vi "Arm Sensors OK.vi"(1 "Motor In":dbl, 2 "Pot Angle":dbl, 3 "Encoder Angle":dbl, 4 "Pot Voltage":dbl) -> (0 "Motor Out":dbl)   [LabVIEW 2013]
uses:
  Robot Global Data.vi
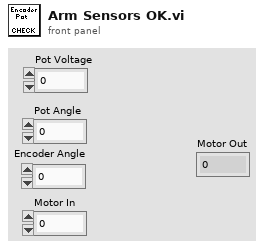
[diagram p1: front panel]
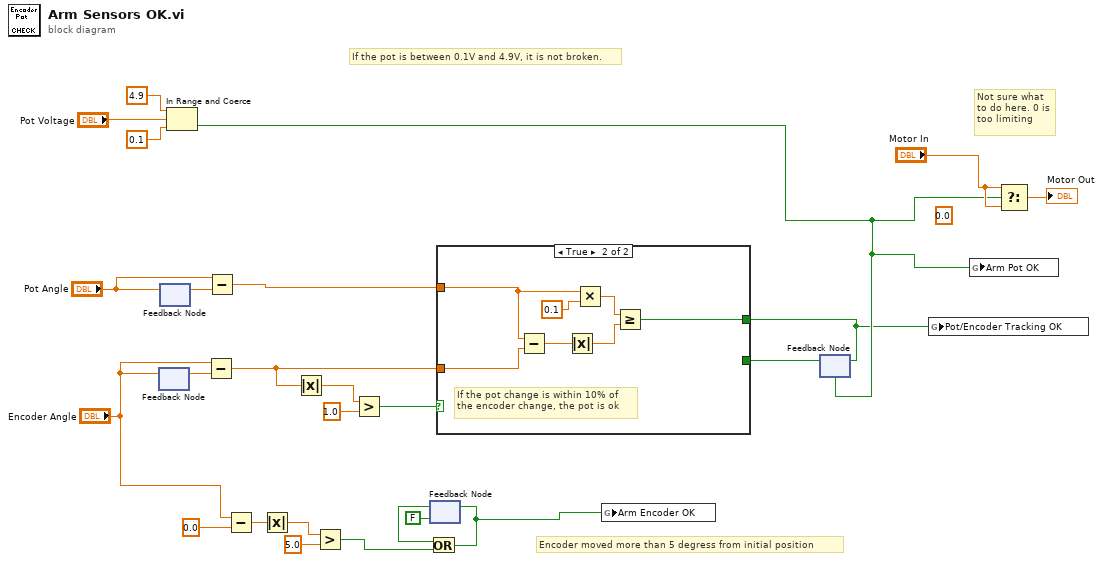
[diagram p0: block diagram]
diagram:
  (unwired) 0.0 ("f")
  # "Not sure what\nto do here. 0 is\ntoo limiting"
  # "Encoder moved more than 5 degress from initial position"
  # "If the pot is between 0.1V and 4.9V, it is not broken."
  n1 = feedback #1() -> (w23:dbl)  [unwired: 1 in]
  n2 = feedback-in #1("Encoder Angle") -> ()
  n3 = feedback #2() -> (w24:dbl)  [unwired: 1 in]
  n4 = feedback-in #2("Pot Angle") -> ()
  n5 = In Range and Coerce(upper limit=4.9 ("y"), x="Pot Voltage", lower limit=0.1 ("y")) -> (In Range?=w2:bool)  [unwired: 1 out]
  n6 = Subtract(x="Encoder Angle", y=w23) -> (x-y=w10:dbl)
  n7 = Subtract(x="Pot Angle", y=w24) -> (x-y=w14:dbl)
  n8 = Subtract(x="Encoder Angle", y=0.0) -> (x-y=w17:dbl)
  n9 = Absolute Value(x=w17) -> (abs(x)=w15:dbl)
  n10 = Absolute Value(x=w10) -> (abs(x)=w11:dbl)
  n11 = Greater?(x=w15, y=5.0) -> (0:w6:bool)
  n12 = Greater?(x=w11, y=1.0) -> (0:w13:bool)
  n13 = feedback #3(FALSE) -> (w5:bool)
  n14 = Or(x=w5, y=w6) -> (x .or. y?=w4:bool)
  n15 = feedback-in #3(w4) -> ()
  n16 = global write "Robot Global Data.vi" "Arm Encoder OK"(w4) -> ()
  n17 = feedback #4(w2) -> (w9:bool)
  n18 = case shown="True" w13 {
    tunnel: w14 -> [_ w28]
    tunnel: w10 -> [_ w29]
    tunnel: [w26 w27] -> w1
    tunnel: w9 -> [w26 _]
    frame False {
    }
    frame True {
      # "If the pot change is within 10% of \nthe encoder change, the pot is ok"
      n19 = Subtract(x=w28, y=w29) -> (x-y=w30:dbl)
      n20 = Absolute Value(x=w30) -> (abs(x)=w32:dbl)
      n21 = Multiply(x=w28, y=0.1) -> (x*y=w33:dbl)
      n22 = Greater Or Equal?(x=w33, y=w32) -> (x >= y?=w27:bool)
    }
  }
  n23 = feedback-in #4(w1) -> ()
  n24 = global write "Robot Global Data.vi" "Pot/Encoder Tracking OK"(w1) -> ()
  n25 = global write "Robot Global Data.vi" "Arm Pot OK"(w2) -> ()
  n26 = Select(t="Motor In", s=w2, f="Motor In") -> (s? t:f=→"Motor Out":dbl)
